vi "Creep Mode.vi"(8 "Drive Input 2":dbl, 9 "Drive Input 1":dbl, 10 "Creep Mode":bool, 11 "Creep Scaler":dbl=0.6) -> (1 "Drive Output 2":dbl, 3 "Drive Output 1":dbl)   [LabVIEW 2012]
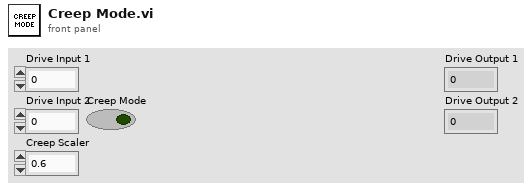
[diagram p1: front panel]
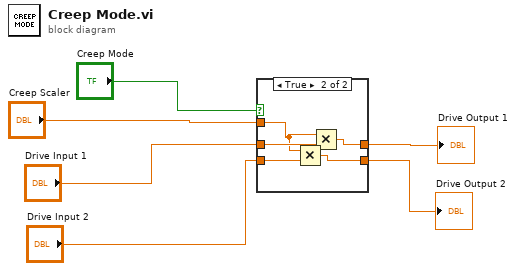
[diagram p0: block diagram]
diagram:
  n1 = case shown="True" "Creep Mode" {
    tunnel: [w7 w10] -> w3
    tunnel: [w8 w11] -> w4
    tunnel: "Drive Input 1" -> [w8 w12]
    tunnel: "Drive Input 2" -> [w7 w13]
    tunnel: "Creep Scaler" -> [_ w9]
    frame False {
    }
    frame True {
      n2 = Multiply(x=w9, y=w13) -> (x*y=w10:dbl)
      n3 = Multiply(x=w9, y=w12) -> (x*y=w11:dbl)
    }
  }
  "Drive Output 1" <- w4
  "Drive Output 2" <- w3
